vi "set_session_id.vi"(0 "control cluster in":T1, 1 "settings in":T2[](array[typedef]) {"stim ramp" min=1}, 2 "setup ID":u16, 3 "error in":errorcluster) -> (7 "control cluster out":T1, 8 "settings out":T2[](array[typedef]) {"stim ramp" min=1}, 9 "Setup ID":i32, 10 "error out":errorcluster)   [LabVIEW 2016]
uses:
  Type Definitions/vars_settings.ctl
  Type Definitions/stim_type.ctl
  Type Definitions/backlight_type.ctl
  Type Definitions/control_references.ctl
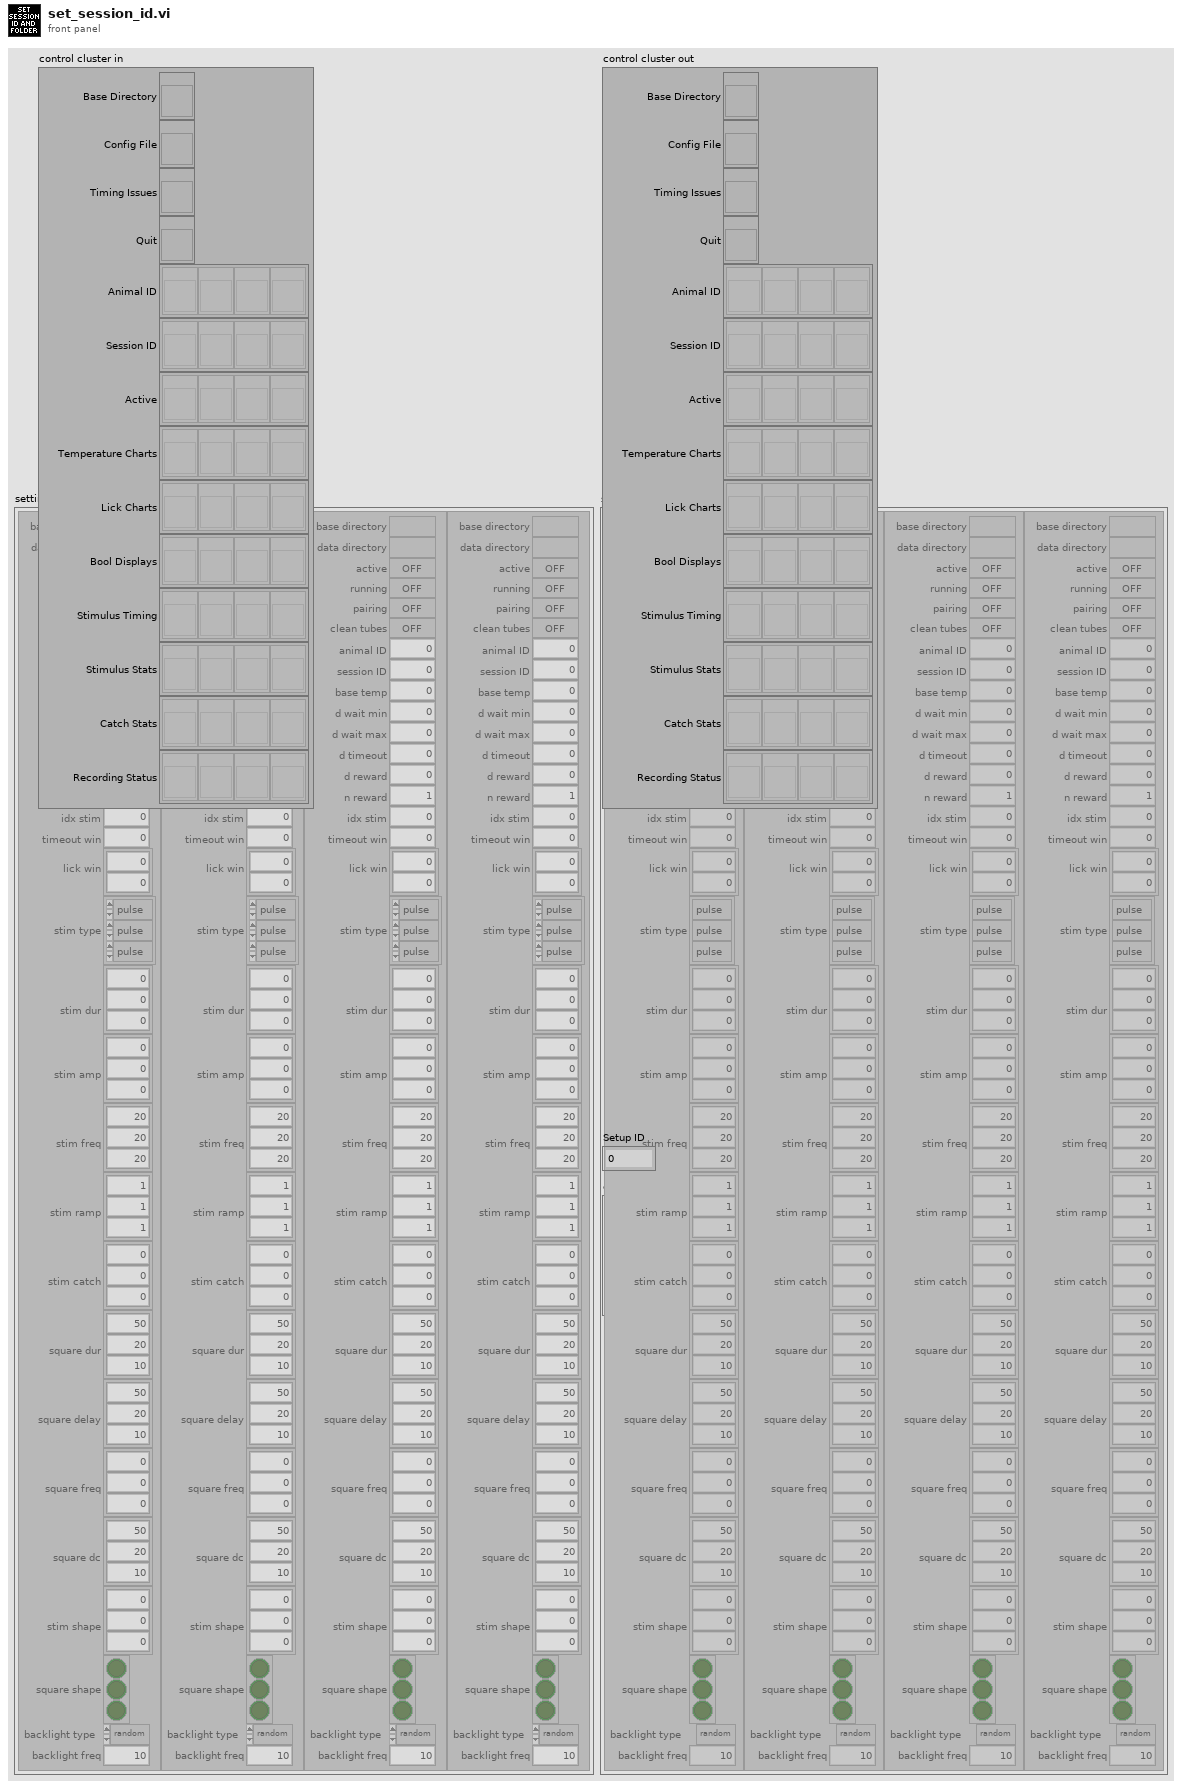
[diagram p1: front panel]
types:
  T1 = typedef "control_references.ctl" = cluster{"Base Directory":refnum<vi>, "Config File":refnum<vi>, "Timing Issues":refnum<vi>, "Quit":refnum<vi>, "Animal ID":refnum<vi>[], "Session ID":refnum<vi>[], "Active":refnum<vi>[], "Temperature Charts":refnum<vi>[], "Lick Charts":refnum<vi>[], "Bool Displays":refnum<vi>[], "Stimulus Timing":refnum<vi>[], "Stimulus Stats":refnum<vi>[], "Catch Stats":refnum<vi>[], "Recording Status":refnum<vi>[]}
  T2 = typedef "vars_settings.ctl" = cluster{"base directory":path, "data directory":path, "active":bool, "running":bool, "pairing":bool, "clean tubes":bool, "animal ID":u16, "session ID":u16, "base temp":dbl, "d wait min":u16, "d wait max":u16, "d timeout":u16, "d reward":u16, "n reward":u16, "idx stim":u16, "timeout win":u16, "lick win":i32[], "stim type":T3[], "stim dur":u16[], "stim amp":dbl[], "stim freq":u16[], "stim ramp":u16[], "stim catch":u8[], "square dur":u16[], "square delay":i16[], "square freq":u8[], "square dc":u8[], "stim shape":dbl[][], "square shape":bool[][], "backlight type":T4, "backlight freq":u16}
  T3 = typedef "stim_type.ctl" = enum16{"pulse", "vibration", "square", "sine"}
  T4 = typedef "backlight_type.ctl" = enum16{"none", "random", "regular"}
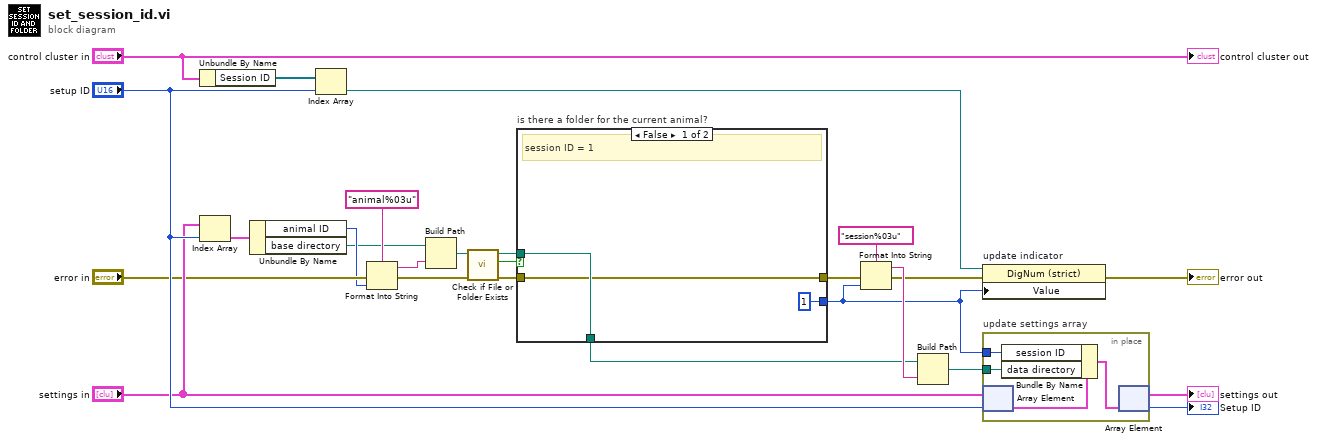
[diagram p0: block diagram]
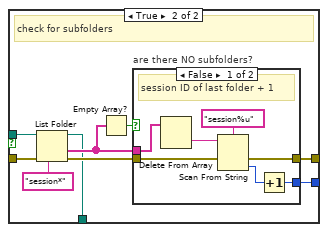
[diagram p2: hidden frame]
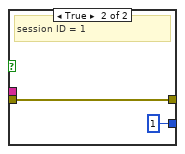
[diagram p3: hidden frame]
diagram:
  n1 = Unbundle By Name("control cluster in") -> ("Session ID"=w18:refnum<vi>[])
  n2 = Index Array(array="settings in", index="setup ID") -> (element=w25:T2)
  n3 = Unbundle By Name(w25) -> ("animal ID"=w15:u16, "base directory"=w14:path)
  n4 = Index Array(array=w18, index="setup ID") -> (element=w16:refnum<vi>)
  n5 = Format Into String(format string="animal%03u" ("pattern"), error in="error in", w15) -> (resulting string=w13:string, error out=w12:errorcluster)  [unwired: 1 in]
  n6 = Build Path(base path=w14, name or relative path=w13) -> (appended path=w11:path)
  n7 = call <vilib>:"Check if File or Folder Exists.vi"("error in (no error)"=w12, "path"=w11) -> ("error out"=w10:errorcluster, "file or folder exists?"=w9:bool, "dup path"=w8:path)  [unwired: 7 in]
  n8 = case "is there a folder for the current animal?" shown="False" w9 {
    tunnel: w10 -> [w28 w37]
    tunnel: [w28 w32] -> w7
    tunnel: w8 -> [w29 w38]
    tunnel: [u32 1 w30] -> w1
    tunnel: [w29 w31] -> w2
    frame False {
      # "session ID = 1"
    }
    frame True {
      # "check for subfolders"
      n9 = List Folder(path=w38, pattern="session*", error in=w37) -> (path out=w31:path, folder names=w34:string[], error out=w33:errorcluster)  [unwired: 1 in, 1 out]
      n10 = Empty Array?(array=w34) -> (empty?=w35:bool)
      n11 = case "are there NO subfolders?" shown="False" w35 {
        tunnel: w34 -> [w45 _]
        tunnel: w33 -> [w43 w47]
        tunnel: [w41 w47] -> w32
        tunnel: [w39 u16 1] -> w30
        frame False {
          # "session ID of last folder + 1"
          n12 = Delete From Array(array=w45) -> (deleted portion=w44:string)  [unwired: 2 in, 1 out]
          n13 = Scan From String(format string="session%u", input string=w44, error in=w43) -> (error out=w41:errorcluster, output 1=w40:u32)  [unwired: 2 in, 2 out]
          n14 = Increment(x=w40) -> (x+1=w39:u32)
        }
        frame True {
          # "session ID = 1"
        }
      }
    }
  }
  n15 = Format Into String(format string="session%03u" ("pattern"), error in=w7, w1) -> (resulting string=w5:string, error out=w4:errorcluster)  [unwired: 1 in]
  n16 = Build Path(base path=w2, name or relative path=w5) -> (appended path=w3:path)
  n17 = property on="update indicator" class="DigNum (strict)"(reference=w16, error in=w4, "Value"=w1) -> (error out=→"error out":errorcluster)  [unwired: 1 out]
  n18 = in-place "update settings array" {
    in-place-border: w3 -> [w51]
    in-place-border: w1 -> [w48]
    n19 = in-place-array #1("settings in", "setup ID") -> (w50:T2)
    n20 = Bundle By Name(cluster=w50, "session ID"=w48, "data directory"=w51) -> (w49:T2)
    n21 = in-place-array #1(w49) -> (→"settings out":T2[], →"Setup ID":i32)
  }
  "control cluster out" <- "control cluster in"
